vi "Cleanup.vi"(8 "error in (no error)":errorcluster, 11 "Endpoint in":refnum<class "Endpoint.lvclass">) -> (0 "error out":errorcluster)   [LabVIEW 2012, in "Stream.lvlib" / "Endpoint.lvclass"]
uses:
  Endpoint.lvclass
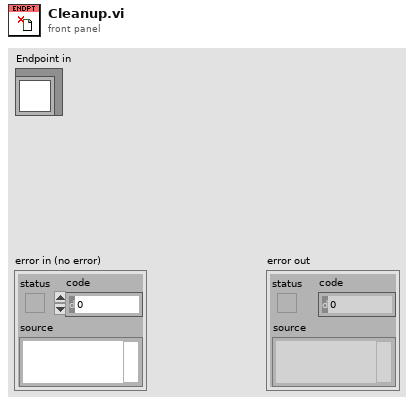
[diagram p1: front panel]
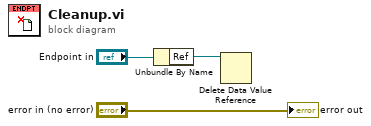
[diagram p0: block diagram]
diagram:
  n1 = Unbundle By Name("Endpoint in") -> ("Ref"=w1:refnum<data-value>)
  n2 = Delete Data Value Reference(data value reference=w1) -> ()  [unwired: 1 in, 2 out]
  "error out" <- "error in (no error)"
